vi "Destroy.vi"(0 "reference in":refnum<class "UI Manager.lvclass">, 5 "Error In":errorcluster) -> (14 "reference out":refnum<class "UI Manager.lvclass">, 19 "Error Out":errorcluster)   [LabVIEW 2024, in "UI Manager.lvclass"]
uses:
  UI Manager.lvclass
  User Manager_class/User Manager.lvclass
  UI Manager.lvclass/UI Manager.ctl
panel:
  # "Connector Pane"
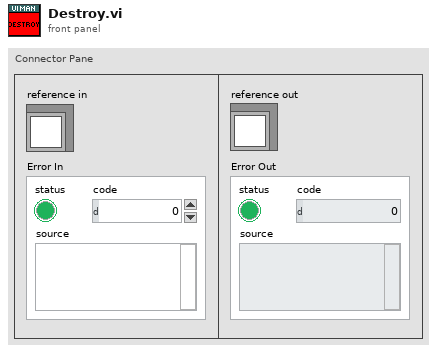
[diagram p1: front panel]
types:
  T1 = typedef "UI Manager.lvclass/ObjectAttributes.ctl" = cluster{"Current Page":refnum<vi>}
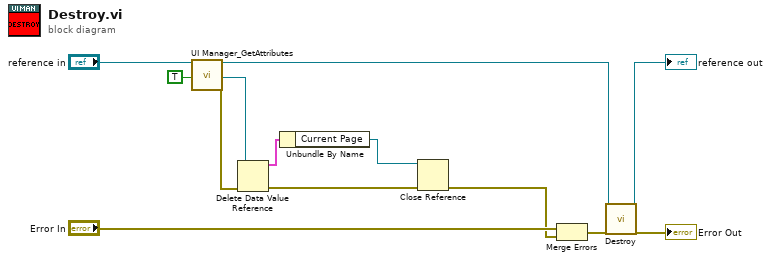
[diagram p0: block diagram]
diagram:
  n1 = call "UI Manager_GetAttributes.vi"("reference in"="reference in", "OnlyGetDvrReference(False)"=TRUE) -> ("reference out"=w8:refnum<class "UI Manager.lvclass">, "DataRef"=w11:refnum<data-value>, "Error Out"=w12:errorcluster)  [unwired: 14 in, 1 out]
  n2 = Delete Data Value Reference(data value reference=w11, error in=w12) -> (data value=w4:T1, error out=w2:errorcluster)
  n3 = Unbundle By Name(w4) -> ("Current Page"=w3:refnum<vi>)
  n4 = Close Reference(reference=w3, error in (no error)=w2) -> (error out=w1:errorcluster)
  n5 = Merge Errors("Error In", w1) -> (w10:errorcluster)
  n6 = call-parent "Destroy.vi"("reference in"=w8, "Error In"=w10) -> ("reference out"=→"reference out":refnum<class "UI Manager.lvclass">, "Error Out"=→"Error Out":errorcluster)  [unwired: 16 in]
